vi "동적장애물.vi"() -> ()   [LabVIEW 2016]
uses:
  <vilib>/imath/engines/lvmath2/RunTimeEngine/Managers/WorkSpace/UID Generator.vi
  <vilib>/imath/engines/lvmath2/RunTimeEngine/IndexRead/NIMS M($,S).vi
  <instcachedir>/0/NIMS M($,S)_3E5749BBB62E49528D4765A77F1F6D98.lvgen/NIMS M($,S)_3E5749BBB62E49528D4765A77F1F6D98_000.vi
  <vilib>/imath/engines/lvmath2/RunTimeEngine/RunTimeType/NIMS_RunTimeType_From StrictType (excl LVString).vi
  <instcachedir>/0/NIMS_RunTimeType_From StrictType (excl LVString)_BBF44FB49F834B71AF7A14CCEDF8BECD.lvgen/NIMS_RunTimeType_From StrictType (excl LVString)_BBF44FB49F834B71AF7A14CCEDF8BECD_000.vi
  <vilib>/imathl/engines/lvmath/Functions/Error Handling/Create Error.vi
  <vilib>/imath/engines/lvmath2/RunTimeEngine/LocalVariableDefStatement/MC_LocalVariableDefStatement_Display.vi
  <vilib>/imath/engines/lvmath2/RunTimeEngine/ArithmeticOperatorToken/NIMS_ArithmeticOperator_plus.vi
  <instcachedir>/0/NIMS_ArithmeticOperator_plus_0120E0498A0F4B4B9BDCAC2554767A4E.lvgen/NIMS_ArithmeticOperator_plus_0120E0498A0F4B4B9BDCAC2554767A4E_004.vi
  <vilib>/imath/engines/lvmath2/RunTimeEngine/BuiltInFunctions/min/1 input/NIMS_min(CV).vi
  <instcachedir>/0/NIMS_min(CV)_95DA9105B87E4BF4B4420F2C454863D6.lvgen/NIMS_min(CV)_95DA9105B87E4BF4B4420F2C454863D6_000.vi
  <vilib>/imath/engines/lvmath2/RunTimeEngine/Managers/SymbolTable/Clear UID.vi
  <vilib>/imath/engines/lvmath2/RunTimeEngine/NodeEndStatement/NIMS_NodeEndStatement_Output.vi
  <instcachedir>/0/NIMS_NodeEndStatement_Output_53EC0D466D134D7ABD903AC30B43404B.lvgen/NIMS_NodeEndStatement_Output_53EC0D466D134D7ABD903AC30B43404B_001.vi
  <vilib>/imath/engines/lvmath2/RunTimeEngine/ErrorHandling/NIMS_Finalize Error.vi
  <vilib>/imath/engines/lvmath2/RunTimeEngine/Managers/SymbolTable/NIMS_WorkSpace.lvlib
panel:
  in  "filter angle(plus)":dbl
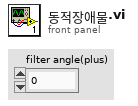
[diagram p1: front panel]
types:
  T1 = typedef "2차원배열 공유변수.ctl" = dbl[][]
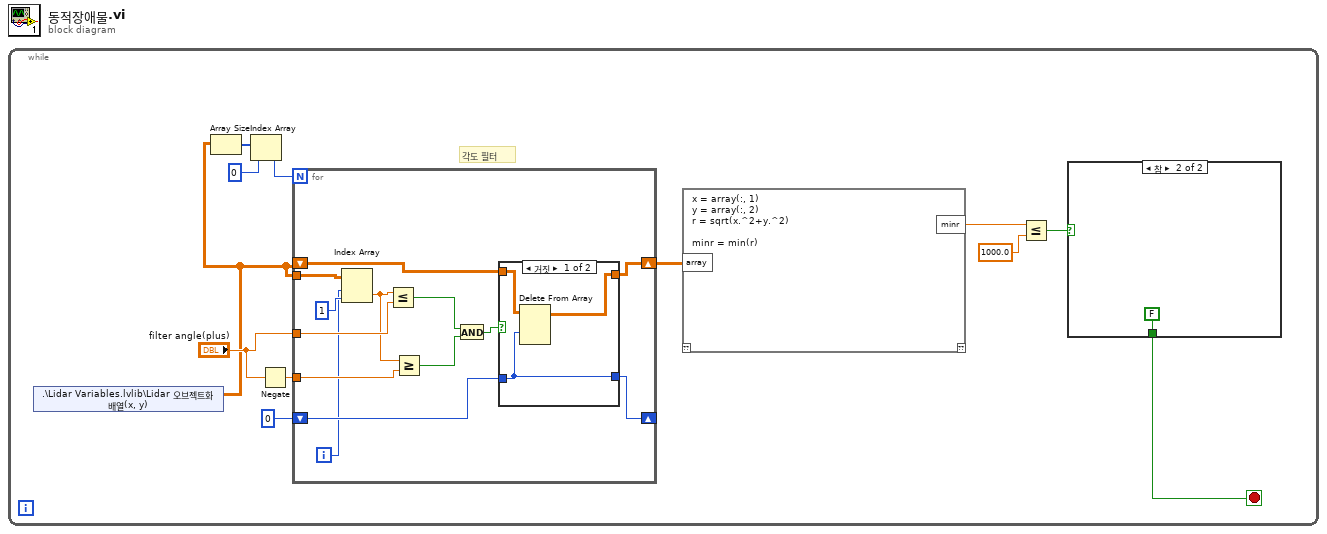
[diagram p0: block diagram]
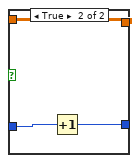
[diagram p2: hidden frame]
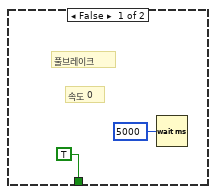
[diagram p3: hidden frame]
diagram:
  n1 = while {
    stop <- w2 stop-if-true
    # "각도 필터"
    n2 = shared-variable ".\\Lidar Variables.lvlib\\Lidar 오브젝트화 배열(x, y)"() -> (w1:T1)  [unwired: 1 in, 1 out]
    n3 = Array Size(array=w1) -> (size(s)=w5:i32[])
    n4 = Index Array(array=w5, index=0 ("인덱스")) -> (element=w3:i32)
    n5 = Negate(x="filter angle(plus)") -> (-x=w8:dbl)
    n6 = for {
      N: w3 -> [_]
      tunnel: "filter angle(plus)" -> [w24]
      tunnel: w8 -> [w22]
      shift-right: [w15] -> _
      shift-left: 0 ("비활성화된 인덱스 (행)") -> [w17]
      shift-right: [w16] -> w6
      shift-left: w1 -> [w18]
      tunnel: w1 -> [w14]
      i -> [w13]
      n7 = Index Array(array=w14, index (row)=w13, index (col)=1 ("비활성화된 인덱스 (열)")) -> (element=w23:dbl)
      n8 = Less Or Equal?(x=w23, y=w24) -> (x <= y?=w21:bool)
      n9 = Greater Or Equal?(x=w23, y=w22) -> (x >= y?=w20:bool)
      n10 = And(x=w21, y=w20) -> (x .and. y?=w19:bool)
      n11 = case shown="거짓" w19 {
        tunnel: w18 -> [w28 w29]
        tunnel: w17 -> [w26 w31]
        tunnel: [w27 w29] -> w16
        tunnel: [w26 w30] -> w15
        frame False {
          n12 = Delete From Array(array=w28, index (row)=w26) -> (array with subset deleted=w27:T1)  [unwired: 2 in, 1 out]
        }
        frame True {
          n13 = Increment(x=w31) -> (x+1=w30:i32)
        }
      }
    }
    n14 = mathscript code="x = array(:, 1)\ny = array(:, 2)\nr = sqrt(x.^2+y.^2)\n\nminr = min(r)"("array"=w6) -> ("minr"=w10:dbl)  [unwired: 1 in, 1 out]
    n15 = Less Or Equal?(x=w10, y=1000.0) -> (x <= y?=w11:bool)
    n16 = case shown="참" w11 {
      tunnel: [TRUE FALSE] -> w2
      frame False {
        # "속도 0"
        # "풀브레이크"
        n17 = Wait (ms)(milliseconds to wait=u32 5000 ("대기 시간 (ms)")) -> ()  [unwired: 1 out]
      }
      frame True {
      }
    }
  }
